vi "CRYData View Legend Manipulate.vi"(6 "Type":enum16{"Curves", "Values", "Results", "WFM"}(ring), 7 "sAction":string, 8 "nData":i32[](array[numeric]), 9 "sData":string, 11 "Legend Ref":refnum<vi>) -> (0 "nData Out":i32[](array[numeric]), 3 "Legend Ref Out":refnum<vi>)   [LabVIEW 2013]
panel:
  in  "Legend":i32[](listbox)
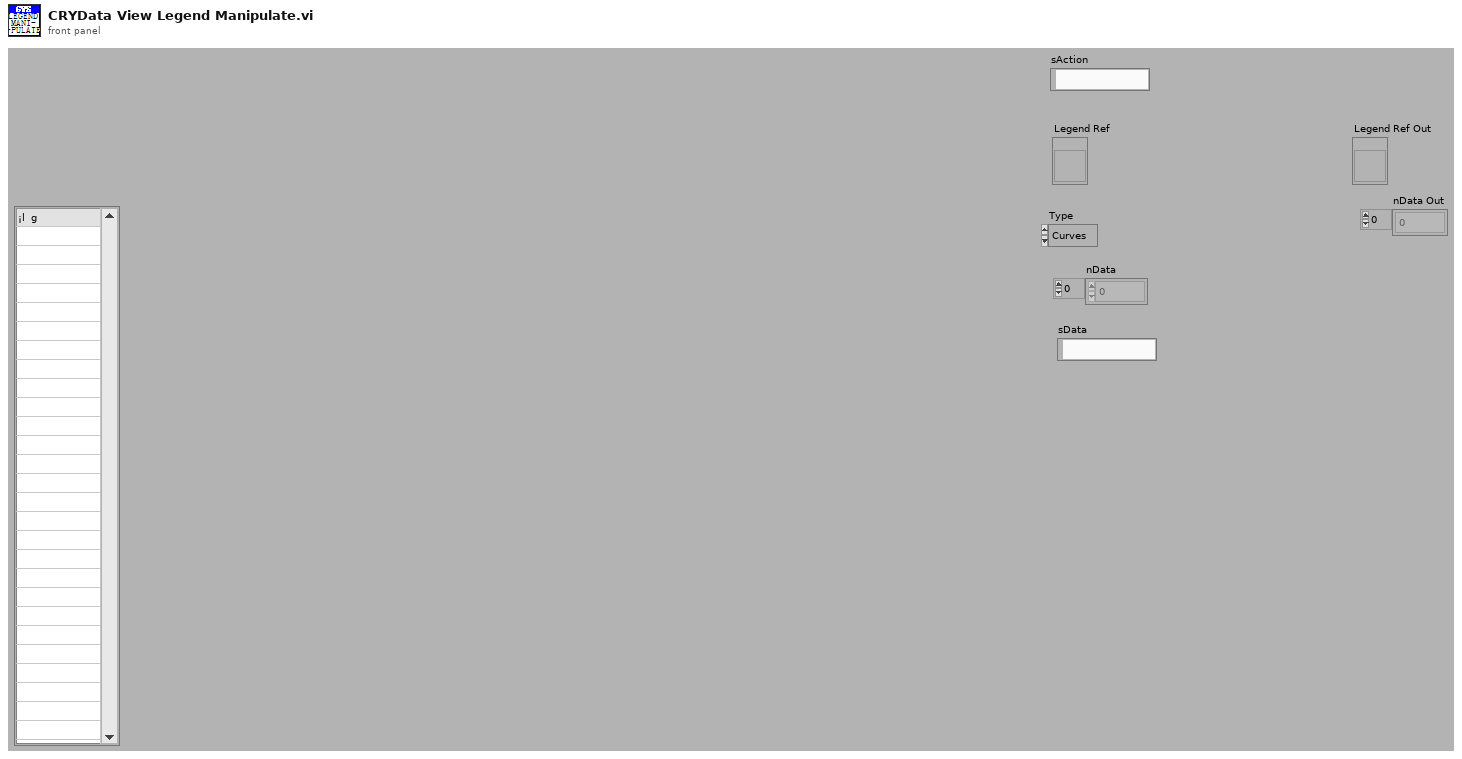
[diagram p1: front panel]
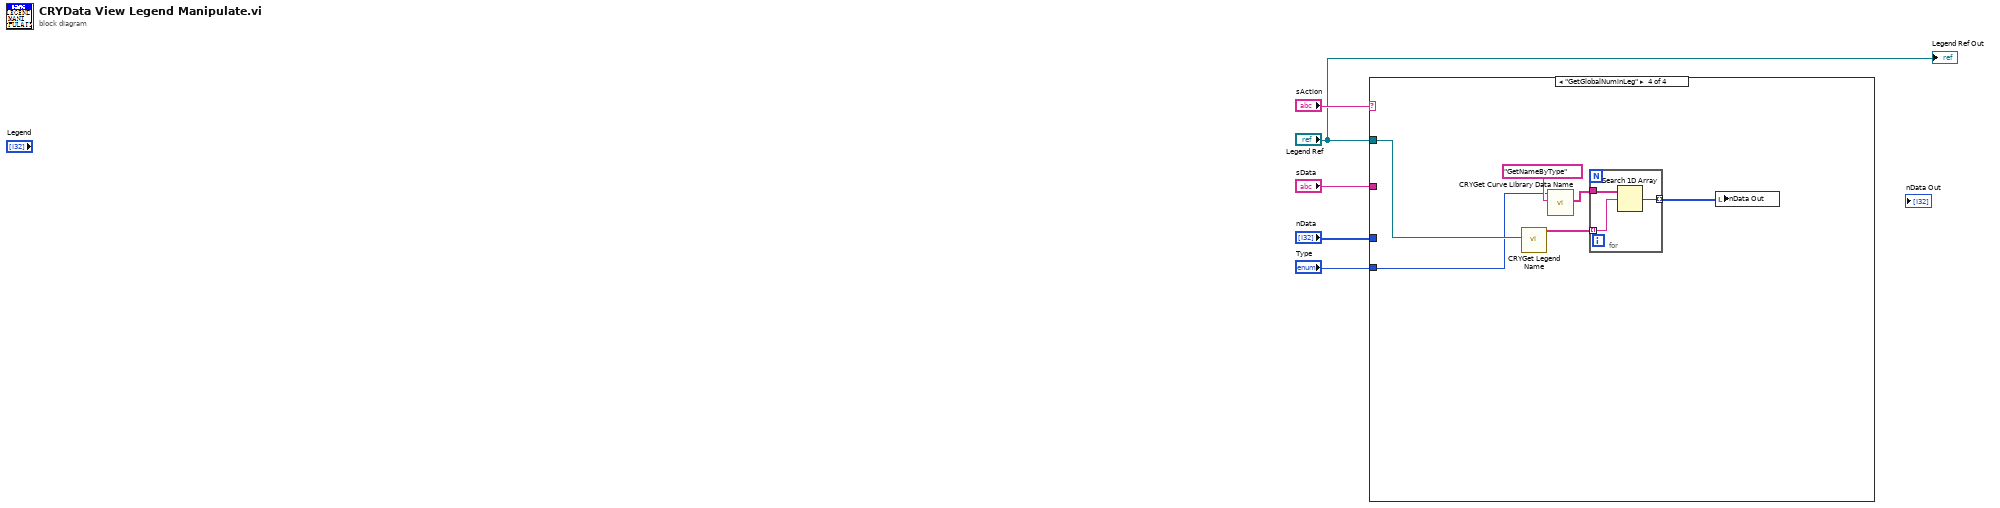
[diagram p0: block diagram]
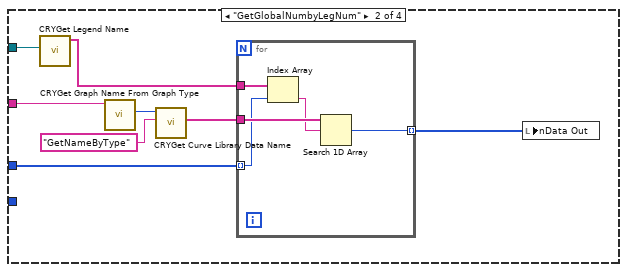
[diagram p3: hidden frame]
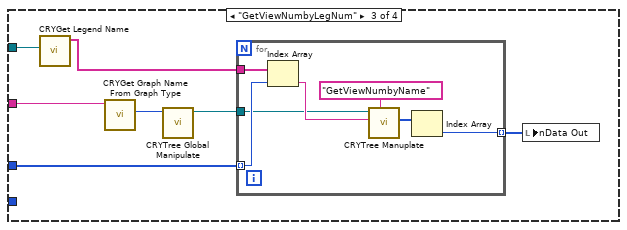
[diagram p4: hidden frame]
diagram:
  n1 = case shown="\"GetGlobalNuminLeg\"" "sAction" {
    tunnel: "sData" -> [_ w9 w24 _]
    tunnel: "nData" -> [_ w6 w21 _]
    tunnel: "Legend Ref" -> [_ w10 w25 w35]
    tunnel: "Type" -> [_ _ _ w33]
    frame Default {
    }
    frame "GetGlobalNumbyLegNum" {
      n2 = call "CRYGet Legend Name.vi"("MCListbox Refnum"=w10) -> ("Names Out"=w8:string[])  [unwired: 10 in]
      n3 = call "CRYGet Graph Name From Graph Type.vi"("Graph Type"=w9) -> ("Type"=w13:enum16{"Curves", "Values", "Results", "WFM"})  [unwired: 9 in, 1 out]
      n4 = call "CRYGet Curve Library Data Name.vi"("sAction"="GetNameByType", "Type"=w13) -> ("sNames"=w11:string[])  [unwired: 6 in, 3 out]
      n5 = for {
        tunnel: w11 -> [w18]
        tunnel: w8 -> [w16]
        tunnel: [w17] -> w7 mode=indexing
        tunnel: w6 -> [w14] mode=indexing
        n6 = Index Array(array=w16, index=w14) -> (element=w15:string)
        n7 = Search 1D Array(1D array=w18, element=w15) -> (index of element=w17:i32)  [unwired: 1 in]
      }
      n8 = local write "nData Out"(w7) -> ()
    }
    frame "GetViewNumbyLegNum" {
      n9 = call "CRYGet Legend Name.vi"("MCListbox Refnum"=w25) -> ("Names Out"=w23:string[])  [unwired: 10 in]
      n10 = call "CRYGet Graph Name From Graph Type.vi"("Graph Type"=w24) -> ("Type"=w20:enum16{"Curves", "Values", "Results", "WFM"})  [unwired: 9 in, 1 out]
      n11 = call "CRYTree Global Manipulate.vi"("Type In"=w20) -> ("Tree/Curve Tree"=w19:refnum<vi>)  [unwired: 7 in, 3 out]
      n12 = for {
        tunnel: w23 -> [w32]
        tunnel: [w27] -> w22 mode=indexing
        tunnel: w21 -> [w31] mode=indexing
        tunnel: w19 -> [w26]
        n13 = Index Array(array=w32, index=w31) -> (element=w29:string)
        n14 = call "CRYTree Manuplate.vi"("sAction"="GetViewNumbyName", "sOption"=w29, "Tree in"=w26) -> ("nData Out"=w28:i32[])  [unwired: 5 in, 3 out]
        n15 = Index Array(array=w28) -> (element=w27:i32)  [unwired: 1 in]
      }
      n16 = local write "nData Out"(w22) -> ()
    }
    frame "GetGlobalNuminLeg" {
      n17 = call "CRYGet Legend Name.vi"("MCListbox Refnum"=w35) -> ("Names Out"=w38:string[])  [unwired: 2 in, 8 out]
      n18 = call "CRYGet Curve Library Data Name.vi"("sAction"="GetNameByType", "Type"=w33) -> ("sNames"=w36:string[])  [unwired: 4 in, 5 out]
      n19 = for {
        tunnel: w36 -> [w41]
        tunnel: w38 -> [w40] mode=indexing
        tunnel: [w39] -> w34 mode=indexing
        n20 = Search 1D Array(1D array=w41, element=w40) -> (index of element=w39:i32)  [unwired: 1 out]
      }
      n21 = local write "nData Out"(w34) -> ()
    }
  }
  "Legend Ref Out" <- "Legend Ref"
